vi "var_num_v0.vi"() -> ()   [LabVIEW 2009]
panel:
  out "Afisare valoare numerica":dbl
  in  "Introducere valoare numerica":dbl
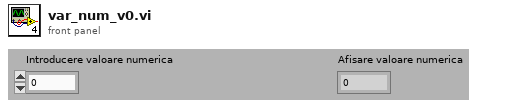
[diagram p1: front panel]
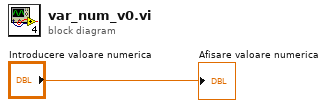
[diagram p0: block diagram]
diagram:
  "Afisare valoare numerica" <- "Introducere valoare numerica"
